vi "TDMS to HDF5.vi"() -> ()   [LabVIEW 2020]
panel:
  out "Channels":string[](array[string])
  out "Groups":string[](array[string])
  in  "TDMS File Path":path
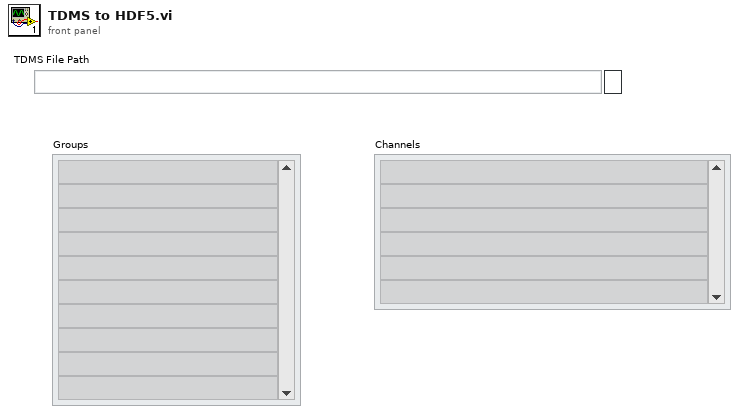
[diagram p1: front panel]
types:
  T1 = enum16{"open", "open or create", "create or replace", "create", "open (read-only)"}
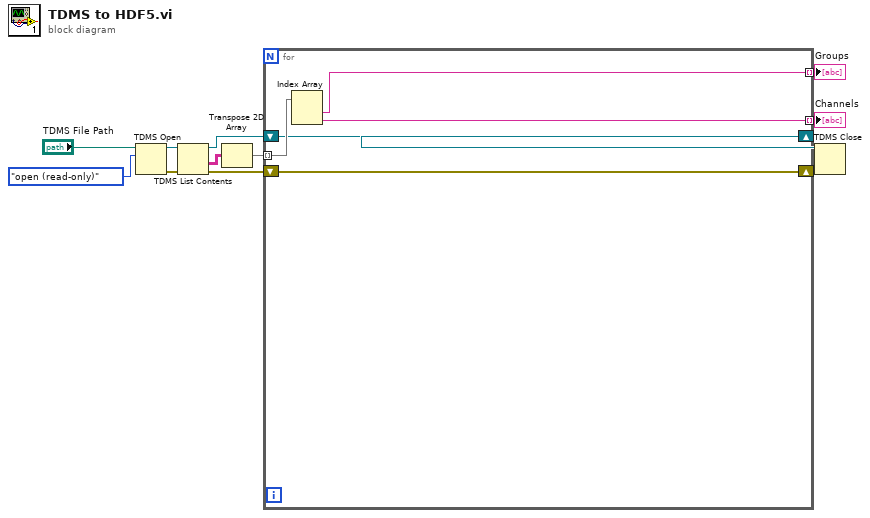
[diagram p0: block diagram]
diagram:
  n1 = TDMS Open(10:T1."open (read-only)" ("operation (0:open)"), 11:"TDMS File Path") -> (0:w10:errorcluster, 3:w11:refnum<k34>)  [unwired: 5 in]
  n2 = TDMS List Contents(4:w10, 7:w11) -> (0:w7:errorcluster, 1:w9:string[][], 3:w8:refnum<k34>)  [unwired: 1 in, 1 out]
  n3 = Transpose 2D Array(2D array=w9) -> (transposed array=w1:string[][])
  n4 = for {
    tunnel: w1 -> [w17] mode=indexing
    shift-right: [w14] -> w6
    shift-left: w8 -> [w14]
    tunnel: [w16] -> w3 mode=indexing
    tunnel: [w15] -> w2 mode=indexing
    shift-right: [w13] -> w5
    shift-left: w7 -> [w13]
    n5 = Index Array(array=w17) -> (element #1=w16:string, element #2=w15:string)  [unwired: 2 in]
  }
  "Groups" <- w3
  "Channels" <- w2
  n6 = TDMS Close(8:w5, 11:w6) -> ()  [unwired: 2 out]
